vi "Amium Kommandos verwalten.vi"(6 "Aktionen":T1, 9 "NEUE Kommandos":string[](array[string])=["ASTZ", "ASTF", "AENT", "ASTZ", "ASTF", "AENT", "ASTZ", "ASTF", "AENT", "ASTF", "ADRU K0 2", "ATEM K0 1", "ATEM K0 2", "ATEM K0 3", "ATEM K0 4", "ATEM K0 5", "ATEM K0 6", "ATEM K0 7", "ATEM K0 8", "ATEM K0 9", "ATEM K0 10", "ATEM K0 11", "ATEM K0 12", "ATEM K0 13", "ATEM K0 14", "ADRU K0 2", "ATES K0 1", "ATES K0 2", "ATES K0 3", "ATES K0 4", "ATES K0 5", "ATES K0 6", "ATES K0 7", "ATES K0 8", "ATES K0 9", "ATES K0 10", "ATES K0 11", "ATES K0 12", "ATES K0 13", "ATES K0 14"], 10 "neues Kommando Array":string[](array[string]), 11 "neues Kommando":string) -> (0 "Zeitstempeln":timestamp[](array[timestamp]), 1 "NEUE Kommandos":string[](array[string])=["ASTZ", "AKON", "AKON", "AKON", "AKON", "AKON", "AKON", "AKON", "AKON", "AKON", "AKON"], 3 "Kommandos":string[](array[string]))   [LabVIEW 2020, in "Amium PNS.lvlib" / "AK Kommunikation.lvlib"]
uses:
  AK Kommunikation.lvlib
  Amium Kommandos verwalten Aktionen.ctl
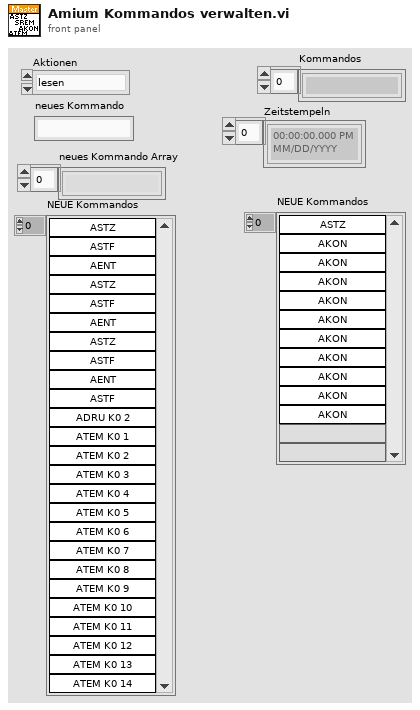
[diagram p1: front panel]
types:
  T1 = typedef "Amium PNS.lvlib/AK Kommunikation.lvlib/Amium Kommandos verwalten Aktionen.ctl" = enum16{"lesen", "setzen Ende", "setzen Pos1", "senden", "initalisieren", "prüfen", "Kommandos"}
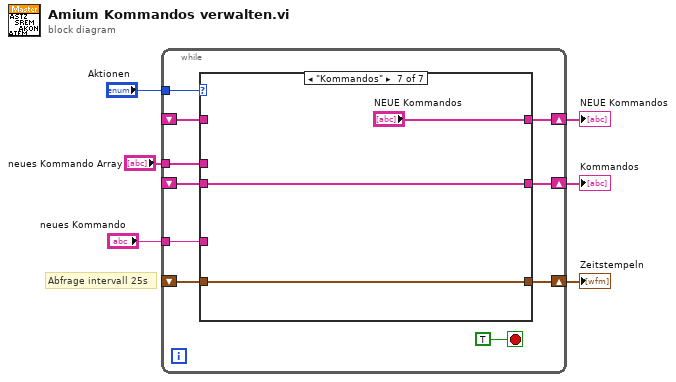
[diagram p0: block diagram]
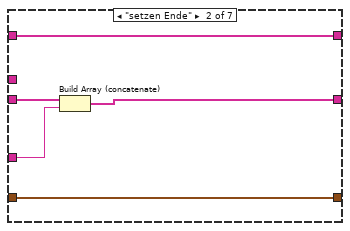
[diagram p3: hidden frame]
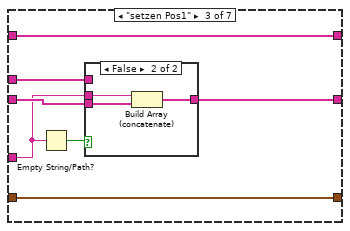
[diagram p4: hidden frame]
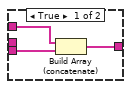
[diagram p5: hidden frame]
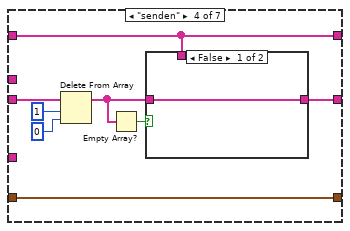
[diagram p6: hidden frame]
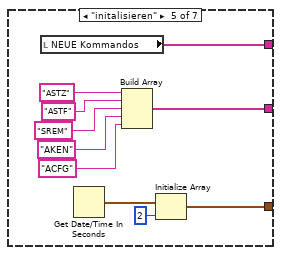
[diagram p8: hidden frame]
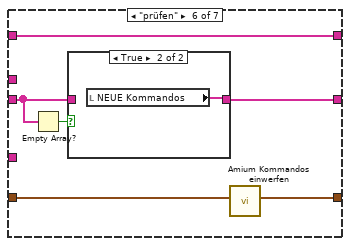
[diagram p9: hidden frame]
diagram:
  # "Abfrage intervall 25s"
  n1 = while {
    tunnel: "Aktionen" -> [w16]
    shift-right: [w14] -> w4
    shift-left: _ -> [w15]
    tunnel: "neues Kommando" -> [w13]
    shift-right: [w11] -> w3
    shift-left: _ -> [w10]
    shift-right: [w9] -> w2
    shift-left: _ -> [w8]
    tunnel: "neues Kommando Array" -> [w7]
    stop <- TRUE stop-if-true
    n2 = case shown="\"Kommandos\"" w16 {
      tunnel: w15 -> [w19 w24 w30 w45 _ w60 w67]
      tunnel: [w19 w23 w29 w39 w54 w58 w67] -> w14
      tunnel: w13 -> [_ w22 w27 _ _ _ _]
      tunnel: [w18 w21 w31 w44 w55 w62 w66] -> w11
      tunnel: w10 -> [w18 w21 w31 w44 _ w63 w66]
      tunnel: [w17 w20 w28 w38 w48 w59 "NEUE Kommandos"] -> w9
      tunnel: w8 -> [w17 w20 w28 w38 _ w59 _]
      tunnel: w7 -> [_ _ w25 _ _ _ _]
      frame "lesen", Default {
      }
      frame "setzen Ende" {
        n3 = Build Array (concatenate)(w24, w22) -> (w23:string[])
      }
      frame "setzen Pos1" {
        n4 = Empty String/Path?(string/path=w27) -> (empty?=w26:bool)
        n5 = case shown="False" w26 {
          tunnel: w30 -> [w34 w37]
          tunnel: [w33 w36] -> w29
          tunnel: w27 -> [_ w35]
          tunnel: w25 -> [w32 _]
          frame True {
            n6 = Build Array (concatenate)(w32, w34) -> (w33:string[])
          }
          frame False {
            n7 = Build Array (concatenate)(w35, w37) -> (w36:string[])
          }
        }
      }
      frame "senden" {
        n8 = Delete From Array(array=w45, length=1 ("Länge"), index=0 ("Index")) -> (array with subset deleted=w40:string[])  [unwired: 1 out]
        n9 = Empty Array?(array=w40) -> (empty?=w41:bool)
        n10 = case shown="False" w41 {
          tunnel: w40 -> [w46 _]
          tunnel: [w46 w47] -> w39
          tunnel: w38 -> [_ w47]
          frame False {
          }
          frame True {
          }
        }
      }
      frame "initalisieren" {
        n11 = local read "NEUE Kommandos"() -> (w48:string[])
        n12 = Get Date/Time In Seconds() -> (seconds since 1Jan1904=w57:timestamp)
        n13 = Build Array("ASTZ", "ASTF", "SREM", "AKEN", "ACFG") -> (w54:string[])
        n14 = Initialize Array(w57, 2 ("Dimension")) -> (w55:timestamp[])
      }
      frame "prüfen" {
        n15 = Empty Array?(array=w60) -> (empty?=w61:bool)
        n16 = case shown="True" w61 {
          tunnel: w60 -> [w64 _]
          tunnel: [w64 w65] -> w58
          frame False {
          }
          frame True {
            n17 = local read "NEUE Kommandos"() -> (w65:string[])
          }
        }
        n18 = call "Amium Kommandos einwerfen.vi"("Zeitstempeln"=w63) -> ("Zeitstempeln"=w62:timestamp[])  [unwired: 9 in, 1 out]
      }
      frame "Kommandos" {
      }
    }
  }
  "Kommandos" <- w4
  "Zeitstempeln" <- w3
  "NEUE Kommandos" <- w2
